vi "CLD 2  Elapsed Time Express FGV Solution.vi"(7 "Timer  Mode":T1, 8 "error in (no error)":errorcluster, 9 "Auto Reset (F)":bool, 11 "Time Target (s)":dbl) -> (0 "error out":errorcluster, 2 "Elapsed Time (s)":dbl format="%#.3g", 3 "Time Has Elapsed":bool)   [LabVIEW 2025]
doc: "CLD 2 exercise\n\nThis SubVI is an FGV that wraps the express VI. \n\nBy default the FGV reset puts False in the auto reset input (and shift register). This occurs only when the \"Set Auto Reset\" case is used. The auto reset must be set as a separate call to the FGV.\n\nIn order to see the functionality this VI must be put into memory. In order to test the FGV a caller VI was created. This is a simple calling VI with a loop, similar to the solution in exercise CLD 1."
uses:
  CLD 2 Time Mode.ctl
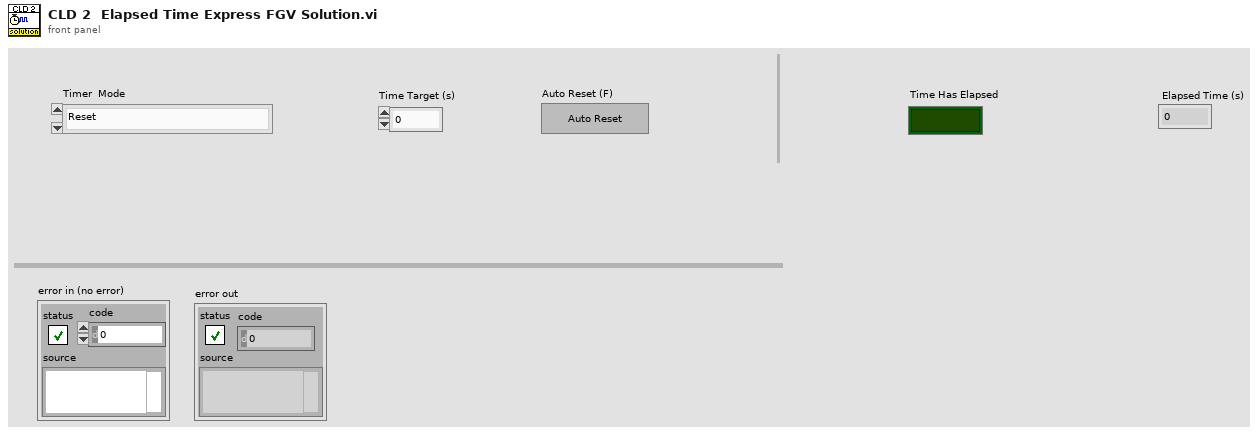
[diagram p1: front panel]
types:
  T1 = typedef "CLD 2 Time Mode.ctl" = enum16{"Reset", "Read Status", "Set Auto Reset"}
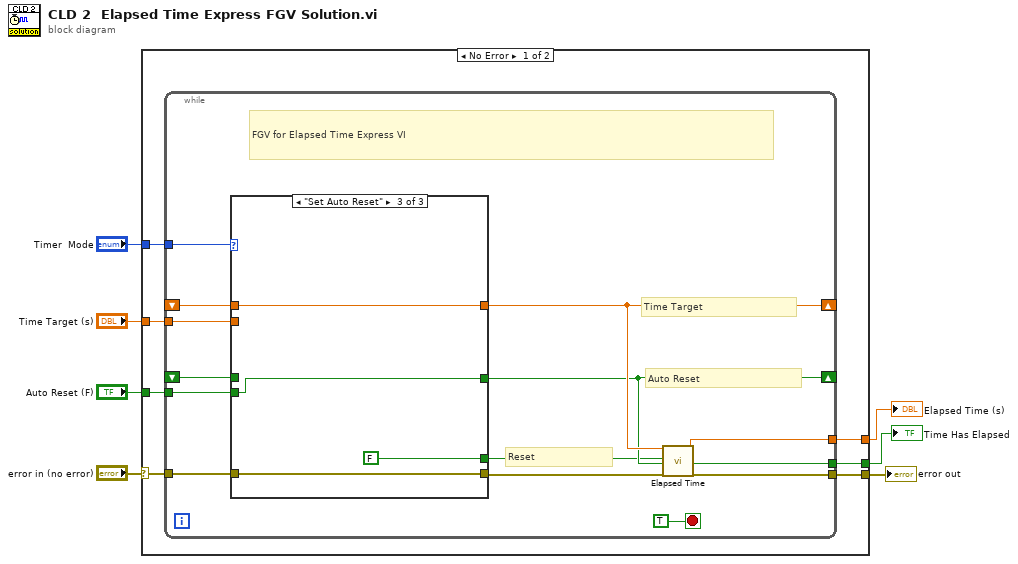
[diagram p0: block diagram]
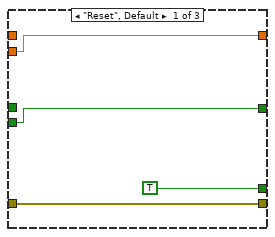
[diagram p2: hidden frame]
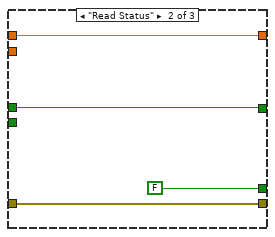
[diagram p3: hidden frame]
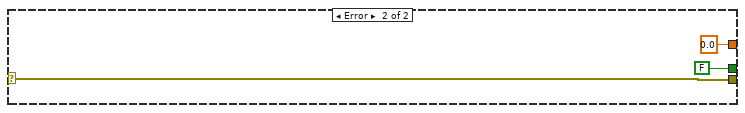
[diagram p4: hidden frame]
diagram:
  n1 = case shown="No Error" "error in (no error)" {
    selector: "error in (no error)" -> [w10 w43]
    tunnel: "Time Target (s)" -> [w14 _]
    tunnel: "Auto Reset (F)" -> [w13 _]
    tunnel: "Timer  Mode" -> [w12 _]
    tunnel: [w11 w43] -> w4
    tunnel: [w9 0.0 ("Elapsed Time (s)")] -> w2
    tunnel: [w8 FALSE ("Time has Elapsed")] -> w1
    frame No Error {
      n2 = while {
        tunnel: w12 -> [w28]
        shift-right: [w25] -> _
        shift-left: _ -> [w27]
        shift-right: [w22] -> _
        shift-left: _ -> [w24]
        tunnel: w14 -> [w26]
        tunnel: w13 -> [w23]
        tunnel: w10 -> [w19]
        tunnel: [w17] -> w11
        tunnel: [w16] -> w9
        tunnel: [w15] -> w8
        stop <- TRUE stop-if-true
        # "Time Target"
        # "Auto Reset"
        # "Reset"
        # "FGV for Elapsed Time Express VI"
        n3 = case shown="\"Set Auto Reset\"" w28 {
          tunnel: w27 -> [_ w36 w40]
          tunnel: [w32 w36 w40] -> w25
          tunnel: w26 -> [w32 _ _]
          tunnel: w24 -> [_ w34 _]
          tunnel: [w31 w34 w39] -> w22
          tunnel: w23 -> [w31 _ w39]
          tunnel: [TRUE FALSE FALSE] -> w21
          tunnel: w19 -> [w29 w33 w37]
          tunnel: [w29 w33 w37] -> w18
          frame "Reset", Default {
          }
          frame "Read Status" {
          }
          frame "Set Auto Reset" {
          }
        }
        n4 = call "Elapsed Time"("Time Target (s)"=w25, "Reset"=w21, "Auto Reset"=w22, "error in (no error)"=w18) -> ("Elapsed Time (s)"=w16:dbl, "Time has Elapsed"=w15:bool, "error out"=w17:errorcluster)  [unwired: 8 in, 5 out]
      }
    }
    frame Error {
    }
  }
  "error out" <- w4
  "Time Has Elapsed" <- w1
  "Elapsed Time (s)" <- w2
